vi "ValidateInput.vi"(8 "error in (no error)":errorcluster, 10 "Input":string, 11 "Code128 in":refnum<class "Code128.lvclass">) -> (0 "error out":errorcluster, 2 "OK":bool=TRUE, 3 "Code128 out":refnum<class "Code128.lvclass">)   [LabVIEW 2013, in "BarCodes.lvlib" / "Code128.lvclass"]
doc: "Returns whether the specified input can be expressed in this barcode format. For this implementation of Code 128, this is whether the text is in the [0-9A-Za-z!\"#$%&'()*+,./:;<=>?A[\\]^_`{|}~-]"
uses:
  Code128.lvclass
  Code128.lvclass/Code128.ctl
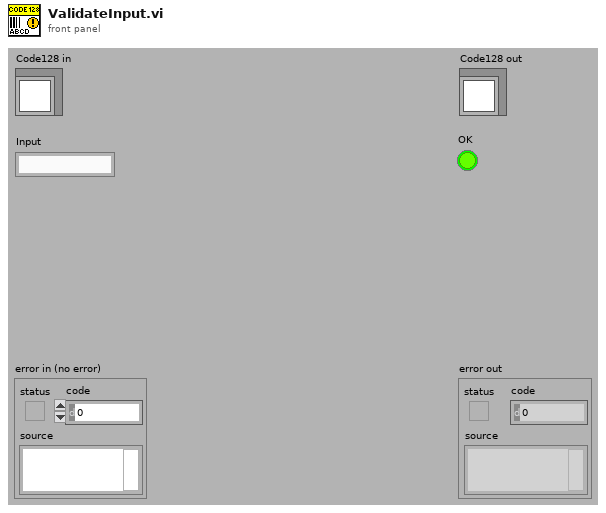
[diagram p1: front panel]
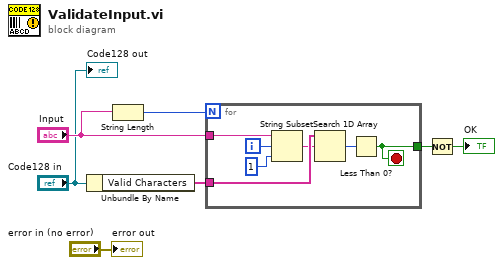
[diagram p0: block diagram]
diagram:
  n1 = Unbundle By Name("Code128 in") -> ("Valid Characters"=w5:string[])
  n2 = String Length(string="Input") -> (length=w7:i32)
  n3 = for {
    N: w7 -> [_]
    tunnel: "Input" -> [w14]
    tunnel: w5 -> [w11]
    tunnel: [w8] -> w4
    i -> [w13]
    stop <- w8 stop-if-true
    n4 = String Subset(string=w14, offset (0)=w13, length (rest)=1 ("length (rest)")) -> (substring=w10:string)
    n5 = Search 1D Array(1D array=w11, element=w10) -> (index of element=w9:i32)  [unwired: 1 in]
    n6 = Less Than 0?(x=w9) -> (x < 0?=w8:bool)
  }
  n7 = Not(x=w4) -> (.not. x?=→"OK":bool)
  "error out" <- "error in (no error)"
  "Code128 out" <- "Code128 in"
